vi "Store Error.vi"(4 "error in (no error)":errorcluster) -> (0 "error out":errorcluster)   [LabVIEW 2015, in "Error Reporting and Storage.lvlib"]
uses:
  Error Reporting and Storage.lvlib
  Standard Signalling/ude_Handle Errors/Event Types.ctl
  Standard Signalling/ude_Handle Errors/ude_Handle Errors.lvlib
  ADO Database Drivers/ADO Database Drivers.lvlib
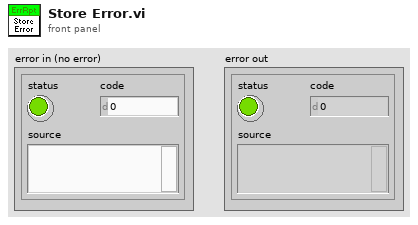
[diagram p1: front panel]
types:
  T1 = typedef "ude_Handle Errors.lvlib/Event Types.ctl" = enum16{"Error", "Warning", "Note"}
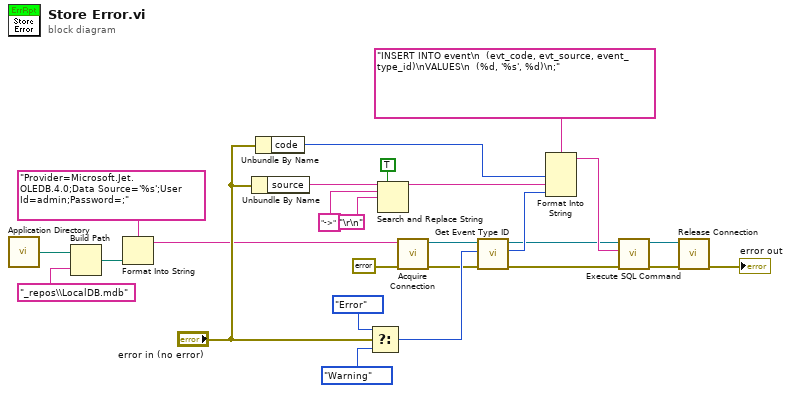
[diagram p0: block diagram]
diagram:
  n1 = call <vilib>:"Application Directory.vi"() -> ("Application Directory"=w7:path)
  n2 = Build Path(base path=w7, name or relative path="_repos\\LocalDB.mdb") -> (appended path=w5:path)
  n3 = Format Into String(format string="Provider=Microsoft.Jet.OLEDB.4.0;Data Source='%s';User Id=admin;Password=;", w5) -> (resulting string=w3:string)  [unwired: 2 in, 1 out]
  n4 = Unbundle By Name("error in (no error)") -> ("source"=w23:string)
  n5 = Unbundle By Name("error in (no error)") -> ("code"=w21:i32)
  n6 = Select(t=Event_Types."Error" ("Event Type"), s="error in (no error)", f=Event_Types."Warning" ("Event Type")) -> (s? t:f=w12:T1)
  n7 = Search and Replace String(replace all?=TRUE ("replace all? (F)"), input string=w23, search string="->", replace string="\r\n") -> (result string=w20:string)  [unwired: 4 in, 3 out]
  n8 = call "Acquire Connection.vi"("error in (no error)"=errorcluster {"status"=FALSE, "code"=0, "source"=""} ("error constant"), "Connection String"=w3) -> ("error out"=w1:errorcluster, "Connection"=w2:refnum<k7>)  [unwired: 3 in, 1 out]
  n9 = call "Get Event Type ID.vi"("error in (no error)"=w1, "Event Type"=w12, "Connection In"=w2) -> ("error out"=w9:errorcluster, "event_type_id"=w11:i32, "Connection Out"=w8:refnum<k7>)  [unwired: 2 in]
  n10 = Format Into String(format string="INSERT INTO event\n  (evt_code, evt_source, event_type_id)\nVALUES\n  (%d, '%s', %d)\n;", w21, w20, w11) -> (resulting string=w17:string)  [unwired: 2 in, 1 out]
  n11 = call "Execute SQL Command.vi"("error in"=w9, "SQL Command"=w17, "Connection In"=w8) -> ("error out"=w19:errorcluster, "Connection Out"=w18:refnum<k7>)  [unwired: 2 in, 1 out]
  n12 = call "Release Connection.vi"("error in"=w19, "Connection"=w18) -> ("error out"=→"error out":errorcluster)  [unwired: 5 in]
